vi "Run Service.vi"(11 "MeasurementLink Server User Events":T1) -> (0 "error out":errorcluster)   [LabVIEW 2024, in "PMIC_Efficiency.lvlib"]
uses:
  PMIC_Efficiency.lvlib
  Advanced/MeasurementPlugin.lvclass
  C:/Program Files/National Instruments/LabVIEW 2024/vi.lib/MeasurementLink/MeasurementLink Measurement Server/Measurement Plugin Service/Measurement Plugin Service.lvclass
  C:/Users/Administrator/Downloads/PMIC_Efficiency/PMIC_Efficiency/Advanced/MeasurementPlugin.lvclass
  <vilib>/MeasurementLink/MeasurementLink Measurement Server/Helpers/TypeDefs/Stop Server User Event.ctl
  <vilib>/MeasurementLink/MeasurementLink Measurement Server/MeasurementLink Measurement Server.lvlib
  <vilib>/MeasurementLink/MeasurementLink Measurement Server/Helpers/TypeDefs/Measurement Service Version.ctl
  <vilib>/MeasurementLink/MeasurementLink Measurement Server/Helpers/TypeDefs/Measurement Server User Settings.ctl
panel:
  # "Run this VI to start the measurement service.  A window will appear that provides basic information about the running service.\n\nUse the stop button on the window that appears to stop the measurement service."
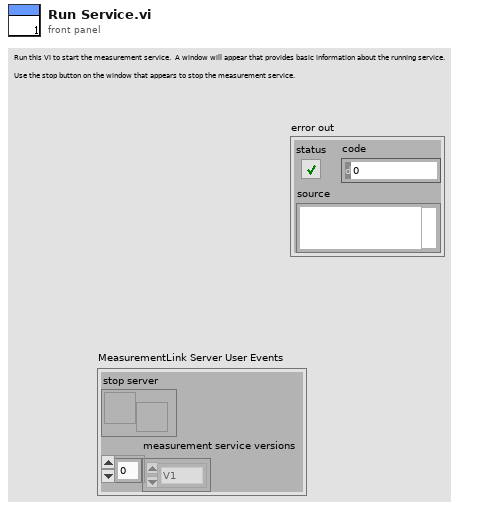
[diagram p1: front panel]
types:
  T1 = typedef "MeasurementLink Measurement Server.lvlib/Measurement Server User Settings.ctl" = cluster{"stop server":T2, "measurement service versions":T3[]}
  T2 = typedef "MeasurementLink Measurement Server.lvlib/Stop Server User Event.ctl" = refnum<user-event>
  T3 = typedef "MeasurementLink Measurement Server.lvlib/Measurement Service Version.ctl" = enum16{"V1", "V2"}
  T4 = enum32{"Invalid", "Standard", "Closed", "Hidden", "Minimized", "Maximized"}
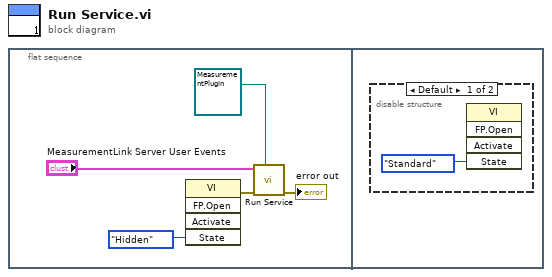
[diagram p0: block diagram]
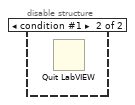
[diagram p2: hidden frame]
diagram:
  n1 = flat-sequence {
    frame #0 {
      n2 = invoke class="VI" method="FP.Open"("State"=T4."Hidden") -> (error out=w3:errorcluster)  [unwired: 4 in, 4 out]
      n3 = call <vilib>:"Run Service.vi"("Measurement"=refnum<class "MeasurementPlugin.lvclass"> refnum ("MeasurementLink Measurement Template.lvlib:Measurement Customizations.lvclass"), "error in (no error)"=w3, "MeasurementLink Server User Events"="MeasurementLink Server User Events") -> ("error out"=→"error out":errorcluster)  [unwired: 8 in]
    }
    frame #1 {
      n4 = disable-structure shown="Default" {
        frame condition #0 (active) {
          n5 = invoke class="VI" method="FP.Open"("State"=T4."Standard") -> ()  [unwired: 4 in, 5 out]
        }
        frame condition #1 {
          n6 = Quit LabVIEW() -> ()  [unwired: 1 in]
        }
      }
    }
  }
